vi "User Validation Check.vi"(7 "Password":string, 8 "error in (no error)":errorcluster, 9 "UserName":string) -> (0 "error out":errorcluster, 2 "FoundUserName":string, 3 "MatchFound?":bool)   [LabVIEW 2024]
uses:
  <vilib>/addons/database/Connection.llb/DB Tools Open Connec (Path).vi
  <vilib>/addons/database/Connection.llb/Conn Execute.vi
  <vilib>/addons/database/Recordset.llb/Rec Fetch Recordset Data (R).vi
  <vilib>/addons/database/Recordset.llb/Rec Destroy - Connection.vi
  <vilib>/addons/database/_DB Variant To Data/Database Variant To Data.xnode
  <vilib>/addons/database/NI_Database_API.lvlib
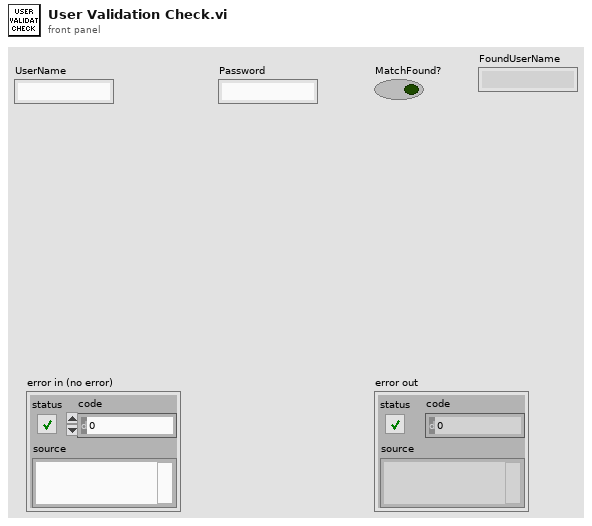
[diagram p1: front panel]
types:
  T1 = typedef "NI_Database_API.lvlib/Conn ObjectReference.ctl" = refnum<k1>
  T2 = typedef "NI_Database_API.lvlib/Rec ObjectReference.ctl" = refnum<k1>
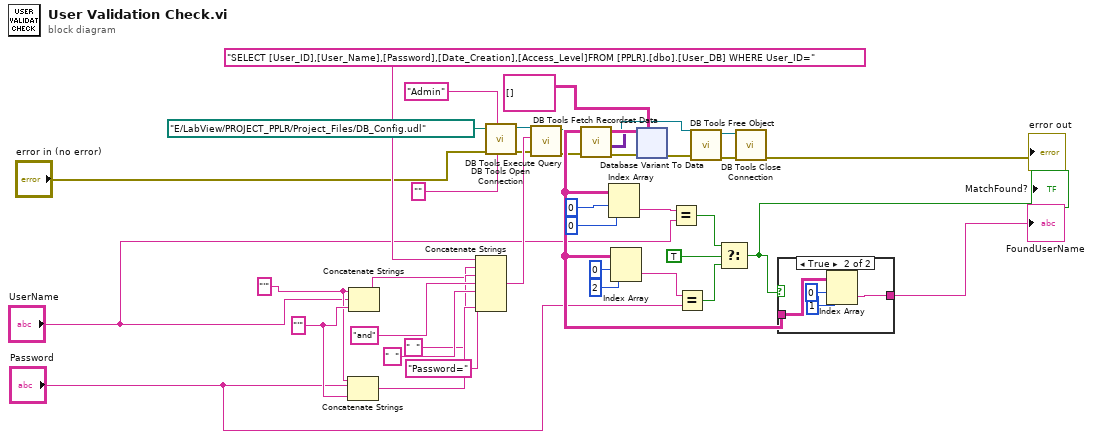
[diagram p0: block diagram]
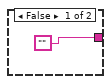
[diagram p2: hidden frame]
diagram:
  w10 = "'"
  w9 = "'"
  n1 = Concatenate Strings(w9, "Password", w10) -> (w16:string)
  n2 = Concatenate Strings(w9, "UserName", w10) -> (w11:string)
  n3 = Concatenate Strings("SELECT [User_ID],[User_Name],[Password],[Date_Creation],[Access_Level]FROM [PPLR].[dbo].[User_DB] WHERE User_ID=", w11, "  " ("string"), "and" ("string"), "  " ("string"), "Password=" ("string"), w16) -> (w17:string)
  n4 = call-poly <vilib>:"DB Tools Open Connection.vi"("password"="", "userID"="Admin", "error in (no error)"="error in (no error)", "connection information"=path "E:/LabView/PROJECT_PPLR/Project_Files/DB_Config.udl" ("File Path")) -> ("error out"=w7:errorcluster, "connection reference"=w6:T1)  [unwired: 4 in]
  n5 = call-poly <vilib>:"DB Tools Execute Query.vi"("error in (no error)"=w7, "SQL query"=w17, "connection reference"=w6) -> ("error out"=w18:errorcluster, "recordset reference"=w19:T2)  [unwired: 5 in]
  n6 = call-poly <vilib>:"DB Tools Fetch Recordset Data.vi"("error in (no error)"=w18, "recordset reference"=w19) -> ("error out"=w20:errorcluster, "recordset data"=w21:variant[][], "recordset reference out"=w23:T2)  [unwired: 3 in]
  n7 = xnode "Database Variant To Data"("database variant"=w21, "error in (no error)"=w20, "type"=string[][] [] ("Array - String")) -> ("data"=w39:string[][], "error out"=w22:errorcluster)
  n8 = Index Array(array=w39, index (row)=0, index (col)=0 ("disabled index (col)")) -> (element=w31:string)
  n9 = Index Array(array=w39, index (row)=0, index (col)=2 ("disabled index (col)")) -> (element=w32:string)
  n10 = Equal?(x=w31, y="UserName") -> (x = y?=w33:bool)
  n11 = Equal?(x=w32, y="Password") -> (x = y?=w34:bool)
  n12 = call-poly <vilib>:"DB Tools Free Object.vi"("error in (no error)"=w22, "recordset reference"=w23) -> ("error out"=w24:errorcluster, "connection reference"=w25:T1)  [unwired: 8 in]
  n13 = Select(t=w33, s=TRUE, f=w34) -> (s? t:f=w38:bool)
  "MatchFound?" <- w38
  n14 = call <vilib>:"DB Tools Close Connection.vi"("error in (no error)"=w24, "connection reference"=w25) -> ("error out"=→"error out":errorcluster)  [unwired: 5 in]
  n15 = case shown="True" w38 {
    tunnel: w39 -> [_ w45]
    tunnel: ["" w42] -> w40
    frame False {
    }
    frame True {
      n16 = Index Array(array=w45, index (row)=0, index (col)=1 ("disabled index (col)")) -> (element=w42:string)
    }
  }
  "FoundUserName" <- w40
